vi "Enqueue.vi"(6 "create if not found? (T)":bool, 7 "Priority (F)":bool, 8 "error in (no error)":errorcluster, 9 "Message Data":variant, 10 "Message":string, 11 "ModuleAdmin":refnum<class "ModuleAdmin.lvclass">) -> (0 "error out":errorcluster, 3 "ModuleAdmin Out":refnum<class "ModuleAdmin.lvclass">)   [LabVIEW 2018, in "SpecAnModule.lvlib"]
doc: "Enqueues a message and message data based on the queue name."
uses:
  SpecAnModule.lvlib
  <userlib>/NIST/ModuleAdminLib/ModuleAdmin/ModuleAdmin.lvclass
  PublicAPI/Arguments/Messages/clMessage.ctl
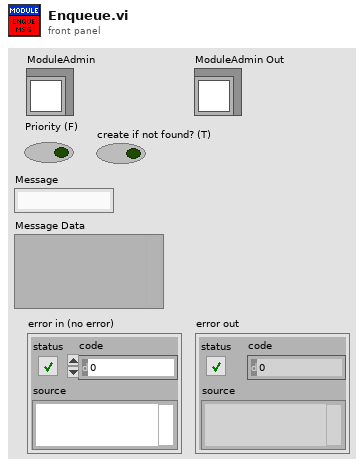
[diagram p1: front panel]
types:
  T1 = typedef "SpecAnModule.lvlib/clMessage.ctl" = cluster{"Message":string, "Message Data":variant}
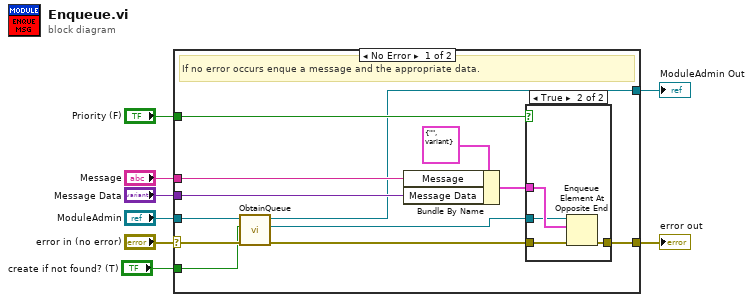
[diagram p0: block diagram]
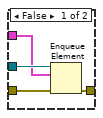
[diagram p2: hidden frame]
diagram:
  n1 = case shown="No Error" "error in (no error)" {
    selector: "error in (no error)" -> [w14 w30]
    tunnel: "Message" -> [w19 _]
    tunnel: "Message Data" -> [w18 _]
    tunnel: "Priority (F)" -> [w17 _]
    tunnel: "ModuleAdmin" -> [w13 w29]
    tunnel: [w16 w30] -> w3
    tunnel: [w10 w29] -> w2
    tunnel: "create if not found? (T)" -> [w9 _]
    frame No Error {
      # "If no error occurs enque a message and the appropriate data."
      n2 = call "ObtainQueue.vi"("error in (no error)"=w14, "create if not found? (f)"=w9, "ModuleAdmin"=w13) -> ("error out"=w12:errorcluster, "queue out"=w11:refnum<queue>, "ModuleAdmin Out"=w10:refnum<class "ModuleAdmin.lvclass">)  [unwired: 6 in]
      n3 = Bundle By Name(cluster=T1 {"Message"="", "Message Data"=variant} ("clMessage"), "Message"=w19, "Message Data"=w18) -> (w20:T1)
      n4 = case shown="True" w17 {
        tunnel: w20 -> [w23 w28]
        tunnel: w11 -> [w24 w27]
        tunnel: [w22 w26] -> w16
        tunnel: w12 -> [w21 w25]
        frame False {
          n5 = Enqueue Element(queue=w24, element=w23, error in (no error)=w21) -> (error out=w22:errorcluster)  [unwired: 1 in, 2 out]
        }
        frame True {
          n6 = Enqueue Element At Opposite End(queue=w27, element=w28, error in (no error)=w25) -> (error out=w26:errorcluster)  [unwired: 1 in, 2 out]
        }
      }
    }
    frame Error {
    }
  }
  "error out" <- w3
  "ModuleAdmin Out" <- w2
